vi "ImageAvailableEventHandler.vi"(4 "User Parameter":variant, 5 "Event Data":cluster{"BufferIndex":i32}, 6 "Control Ref":refnum<k7>, 7 "Event Common Data":T1) -> ()   [LabVIEW 2017]
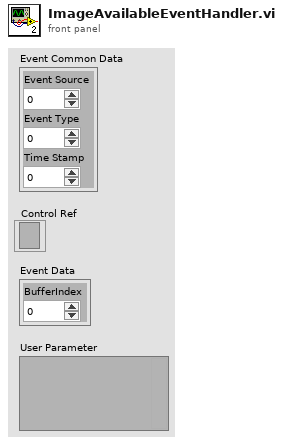
[diagram p1: front panel]
types:
  T1 = cluster{"Event Source":i32, "Event Type":u32, "Time Stamp":u32}
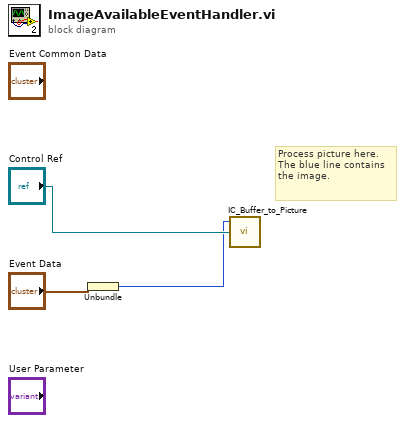
[diagram p0: block diagram]
diagram:
  # "Process picture here. The blue line contains the image."
  n1 = Unbundle("Event Data") -> ("BufferIndex"=w1:i32)
  n2 = call "IC_Buffer_to_Picture.vi"("Item"=w1, "ICImagingControl In"="Control Ref") -> ()  [unwired: 1 in, 4 out]
